vi "Read Element of Sounds.vi"(10 "index":i32, 11 "Aggregate Sound in":refnum<class "Aggregate Sound.lvclass">) -> (2 "Sound.lvclass":refnum<class "Sound.lvclass">, 3 "Aggregate Sound out":refnum<class "Aggregate Sound.lvclass">)   [LabVIEW 2010, in "Aggregate Sound.lvclass"]
uses:
  Aggregate Sound.lvclass
  Sound/Sound.lvclass
  Aggregate Sound.lvclass/Aggregate Sound.ctl
  Silence/Silence.lvclass
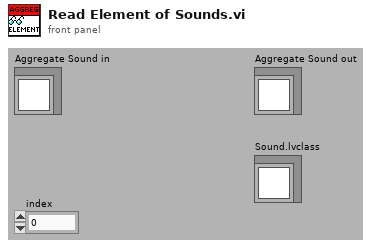
[diagram p1: front panel]
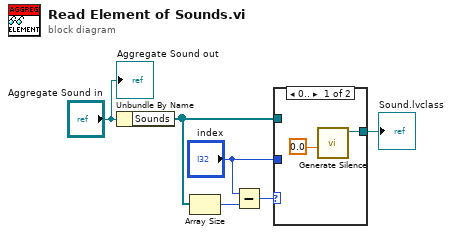
[diagram p0: block diagram]
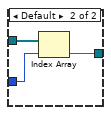
[diagram p2: hidden frame]
diagram:
  n1 = Unbundle By Name("Aggregate Sound in") -> ("Sounds"=w4:refnum<class "Sound.lvclass">[])
  n2 = Array Size(array=w4) -> (size(s)=w2:i32)
  n3 = Subtract(x="index", y=w2) -> (x-y=w1:i32)
  n4 = case shown="0.." w1 {
    tunnel: [w7 w11] -> w5
    tunnel: w4 -> [_ w10]
    tunnel: "index" -> [_ w9]
    frame 0.. {
      n5 = call "Generate Silence.vi"("Duration (1 second)"=0.0) -> ("Silence out"=w7:refnum<class "Silence.lvclass">)  [unwired: 10 in]
    }
    frame Default {
      n6 = Index Array(array=w10, index=w9) -> (element=w11:refnum<class "Sound.lvclass">)
    }
  }
  "Sound.lvclass" <- w5
  "Aggregate Sound out" <- "Aggregate Sound in"
